vi "Update DSM Level.vi"() -> (3 "DSM Message":string)   [LabVIEW 2016]
uses:
  Custom Pallet Controls/Custom Pallet Forward.ctl
panel:
  in  "DSM Level":T1(ring)
  out "Description":string="Update DSM Level"
  in  "Complete":T2
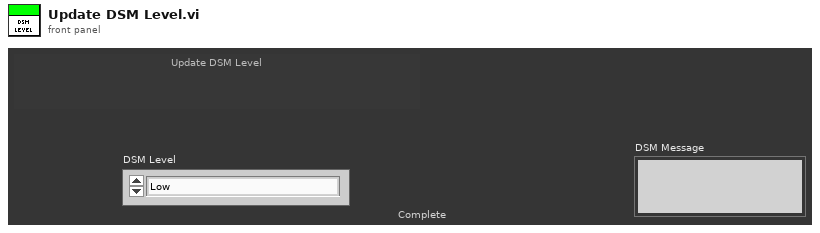
[diagram p1: front panel]
types:
  T1 = enum16{"Low", "Medium", "High", "Very High", "Critical"}
  T2 = typedef "Custom Pallet Forward.ctl" = bool
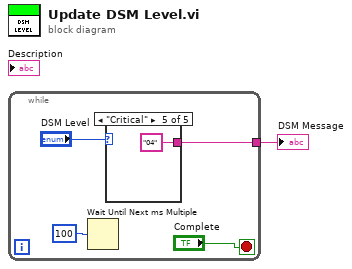
[diagram p0: block diagram]
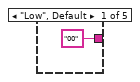
[diagram p2: hidden frame]
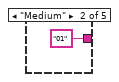
[diagram p3: hidden frame]
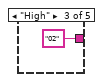
[diagram p4: hidden frame]
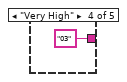
[diagram p5: hidden frame]
diagram:
  n1 = while {
    tunnel: [w2] -> w1
    stop <- "Complete" stop-if-true
    n2 = Wait Until Next ms Multiple(millisecond multiple=u32 100) -> ()  [unwired: 1 out]
    n3 = case shown="\"Critical\"" "DSM Level" {
      tunnel: ["00" "01" "02" "03" "04"] -> w2
      frame "Low", Default {
      }
      frame "Medium" {
      }
      frame "High" {
      }
      frame "Very High" {
      }
      frame "Critical" {
      }
    }
  }
  "DSM Message" <- w1
